vi "geve-init_com_refs.vi"(8 "error in (no error)":errorcluster) -> (0 "error out":errorcluster, 3 "com-refs":T1)   [LabVIEW 2018]
doc: "creates applications coms refs."
uses:
  geve-com_ref_cluster.ctl
  geve-message_cluster.ctl
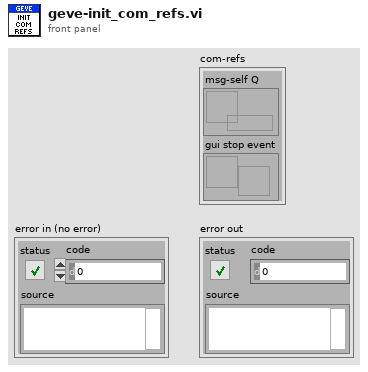
[diagram p1: front panel]
types:
  T1 = typedef "geve-com_ref_cluster.ctl" = cluster{"msg-self Q":refnum<queue>, "gui stop event":refnum<user-event>}
  T2 = typedef "geve-message_cluster.ctl" = cluster{"Command":string, "Payload":variant}
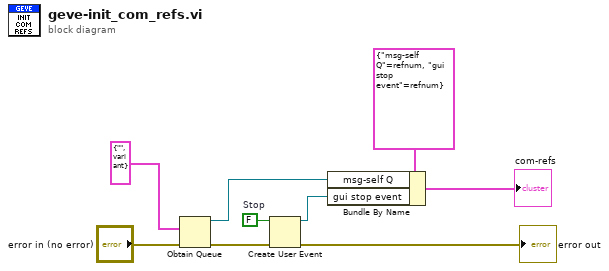
[diagram p0: block diagram]
diagram:
  w4 = FALSE  # Stop
  n1 = Obtain Queue(element data type=T2 {"Command"="", "Payload"=variant} ("Message"), error in (no error)="error in (no error)") -> (queue out=w1:refnum<queue>, error out=w7:errorcluster)  [unwired: 3 in, 1 out]
  n2 = Create User Event(user event datatype=w4, error in=w7) -> (user event=w6:refnum<user-event>, error out=→"error out":errorcluster)
  n3 = Bundle By Name(cluster=T1 {"msg-self Q"=refnum, "gui stop event"=refnum} ("com-refs"), "msg-self Q"=w1, "gui stop event"=w6) -> (→"com-refs":T1)
